vi "Test Filter Dashed Class in Library.vi"(8 "error in (no error)":errorcluster, 11 "Test Case In":refnum<class "Filter Test.lvclass">) -> (0 "error out":errorcluster, 3 "Test Case Out":refnum<class "Filter Test.lvclass">)   [LabVIEW 2020, in "Filter Test.lvclass"]
uses:
  Filter Test.lvclass
  C:/Program Files (x86)/National Instruments/LabVIEW 2020/vi.lib/Astemes/LUnit/Test Case.lvclass
  <vilib>/Astemes/LUnit/Test Case.lvclass/Test Case.ctl
  <vilib>/Astemes/LUnit/Append Fail Result.vi
  <vilib>/Astemes/LUnit/Append Pass Result.vi
  source/Support/Filters/Dashed Filter/Dashed Filter.lvclass
  Filter Test.lvclass/Filter Test.ctl
  source/API/LUnit Test Suite/LUnit Test Suite.lvclass
  <vilib>/Astemes/LUnit/Test Case.lvclass
panel:
  out "List of Runnables":string[](array[string])
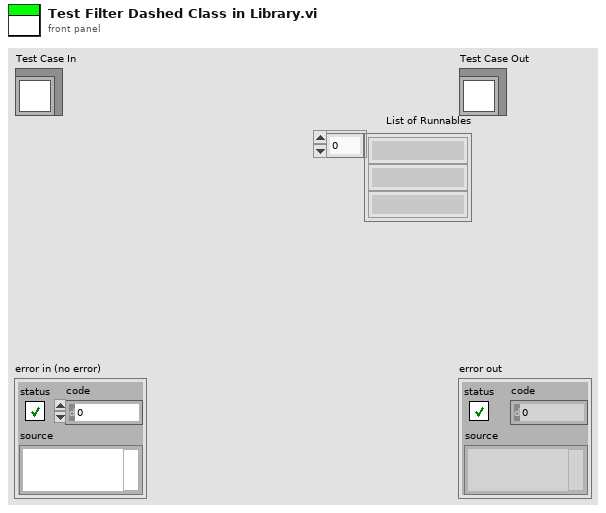
[diagram p1: front panel]
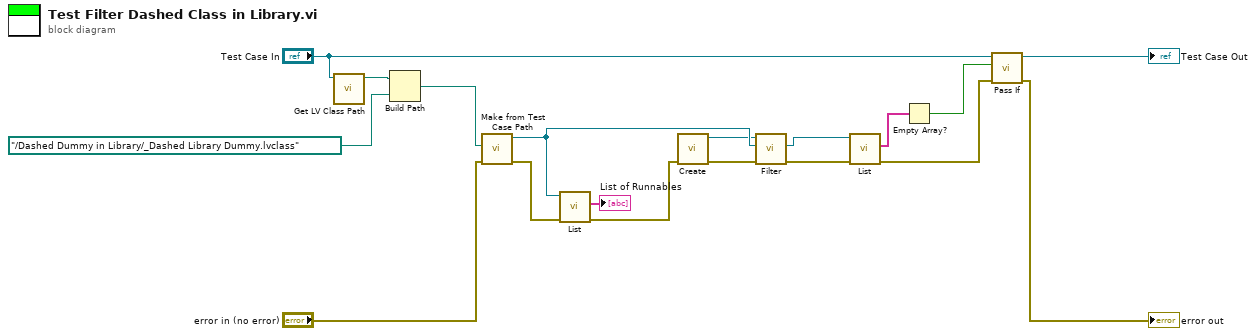
[diagram p0: block diagram]
diagram:
  n1 = call <vilib>:"Get LV Class Path.vi"("object"="Test Case In") -> ("class path"=w9:path)  [unwired: 9 in, 1 out]
  n2 = Build Path(base path=w9, name or relative path=path "../Dashed Dummy in Library/_Dashed Library Dummy.lvclass") -> (appended path=w7:path)
  n3 = call "Make from Test Case Path.vi"("error in (no error)"="error in (no error)", "Test Case"=w7) -> ("error out"=w16:errorcluster, "LUnit Test Suite Out"=w11:refnum<class "LUnit Test Suite.lvclass">)  [unwired: 8 in]
  n4 = call "List.vi"("error in (no error)"=w16, "LUnit Test Suite In"=w11) -> ("error out"=w5:errorcluster, "List of Runnables"=→"List of Runnables":string[])  [unwired: 8 in]
  n5 = call "Create.vi"("error in (no error)"=w5) -> ("error out"=w4:errorcluster, "Dashed Filter"=w6:refnum<class "Dashed Filter.lvclass">)  [unwired: 9 in]
  n6 = call-dynamic "Filter.vi"("error in (no error)"=w4, "Test Suite"=w11, "Dashed Filter in"=w6) -> ("error out"=w14:errorcluster, "Filtered Test Suite"=w15:refnum<class "LUnit Test Suite.lvclass">)  [unwired: 7 in]
  n7 = call "List.vi"("error in (no error)"=w14, "LUnit Test Suite In"=w15) -> ("error out"=w13:errorcluster, "List of Runnables"=w3:string[])  [unwired: 8 in]
  n8 = Empty Array?(array=w3) -> (empty?=w2:bool)
  n9 = call <vilib>:"Pass If.vi"("error in (no error)"=w13, "Pass?"=w2, "LUnit Test Case In"="Test Case In") -> ("error out"=→"error out":errorcluster, "LUnit Test Case Out"=→"Test Case Out":refnum<class "Filter Test.lvclass">)  [unwired: 7 in]
